vi "steerdrive.vi"() -> ()   [LabVIEW 2014, in "Janga.lvrbt"]
uses:
  Janga.lvrbt
  <vilib>/NXT/LegoClasses/BrickReference/BrickReference.lvclass
  <vilib>/NXT/Subs/LVHSConnector.ctl
  <vilib>/NXT/NXTIO Xnodes/NXTIOXNode/NXTIO.xnode
  <vilib>/NXT/Block Support/NXT_OutputPort.ctl
  <vilib>/NXT/NXTIO Xnodes/AddressXNode/NXTIOAddress.xnode
  <vilib>/NXT/NXTIO Xnodes/NXTIONodeSubVIs/NXTStopMotors.vi
  <vilib>/NXT/Subs/MotorOutput.ctl
panel:
  in  "Amount":i32=100
  in  "Steering (100)":i32=100
  in  "Power (75)":i32=75
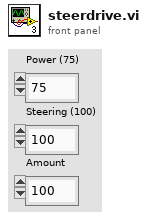
[diagram p1: front panel]
types:
  T1 = typedef "NXT_OutputPort.ctl" = u8
  T2 = typedef "MotorOutput.ctl" = u8
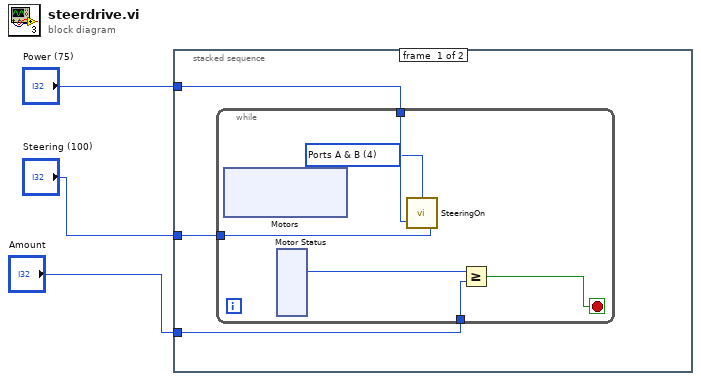
[diagram p0: block diagram]
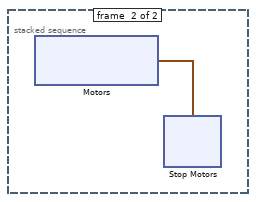
[diagram p2: hidden frame]
diagram:
  n1 = stacked-sequence {
    tunnel: "Power (75)" -> [w6 _]
    tunnel: "Steering (100)" -> [w5 _]
    tunnel: "Amount" -> [w4 _]
    frame #0 {
      n2 = while {
        tunnel: w6 -> [w12]
        tunnel: w5 -> [w11]
        tunnel: w4 -> [w9]
        stop <- w8 stop-if-true
        w7 = T2 4 items=["Port A"=0, "Port B"=1, "Port C"=2, "Ports A & B"=4, "Ports A & C"=5, "Ports B & C"=6, "All Ports"=3] ("Output Ports (A & B)")
        n3 = xnode "Motors"() -> ()  [unwired: 1 out]
        n4 = xnode "Motor Status"() -> ("Position 1"=w10:i32)  [unwired: 2 in, 2 out]
        n5 = call <vilib>:"SteeringOn.vi"("Power (75)"=w12, "Steering (100)"=w11, "Output Ports (A & B)"=w7) -> ()  [unwired: 1 in, 1 out]
        n6 = Greater Or Equal?(x=w10, y=w9) -> (x >= y?=w8:bool)
      }
    }
    frame #1 {
      n7 = xnode "Motors"() -> ("Motor"=w14:cluster{"Port":T1, "Port":T1})
      n8 = xnode "Stop Motors"("Motors"=w14) -> ()  [unwired: 1 in, 1 out]
    }
  }
